vi "Open Camera.vi"(8 "error in (no error)":errorcluster) -> (0 "error out":errorcluster, 3 "Camera":refnum<data-value>)   [LabVIEW 2020, in "Test.Camera.lvclass"]
uses:
  Test.Camera.lvclass
  g_industrial_cam/Camera/Camera.lvclass
  Test.Camera.lvclass/Test.Camera.ctl
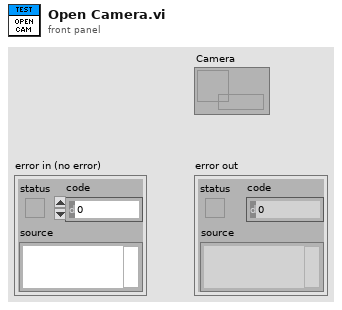
[diagram p1: front panel]
types:
  T1 = typedef "Device Enumeration.ctl" = cluster{"ID":string, "Protocol":string, "Vendor":string, "Model":string, "Serial":string, "Address":string}
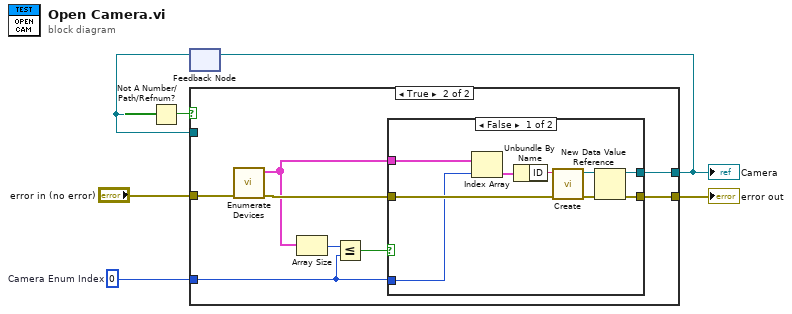
[diagram p0: block diagram]
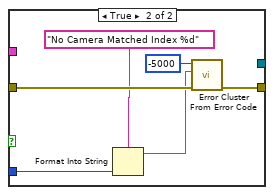
[diagram p3: hidden frame]
diagram:
  w1 = 0  # Camera Enum Index
  n1 = feedback #1() -> (w2:refnum<data-value>)  [unwired: 1 in]
  n2 = Not A Number/Path/Refnum?(number/path/refnum=w2) -> (NaN/Path/Refnum?=w3:bool)
  n3 = case shown="True" w3 {
    tunnel: "error in (no error)" -> [w8 w16]
    tunnel: [w8 w14] -> w5
    tunnel: [w7 w13] -> w4
    tunnel: w2 -> [w7 _]
    tunnel: w1 -> [_ w10]
    frame False {
    }
    frame True {
      n4 = call "Enumerate Devices.vi"("error in (no error)"=w16) -> ("error out"=w15:errorcluster, "Devices"=w12:T1[])  [unwired: 9 in]
      n5 = Array Size(array=w12) -> (size(s)=w11:i32)
      n6 = Less Or Equal?(x=w11, y=w10) -> (x <= y?=w9:bool)
      n7 = case shown="False" w9 {
        tunnel: w15 -> [w24 w31]
        tunnel: w10 -> [w22 w28]
        tunnel: [w20 w30] -> w14
        tunnel: [w18 _] -> w13
        tunnel: w12 -> [w17 _]
        frame False {
          n8 = Index Array(array=w17, index=w22) -> (element=w21:T1)
          n9 = Unbundle By Name(w21) -> ("ID"=w25:string)
          n10 = call "Create.vi"("error in (no error)"=w24, "Identifier (ID, IP etc)"=w25) -> ("error out"=w23:errorcluster, "Camera"=w19:refnum<class "Camera.lvclass">)  [unwired: 8 in]
          n11 = New Data Value Reference(data value=w19, error in=w23) -> (data value reference=w18:refnum<data-value>, error out=w20:errorcluster)
        }
        frame True {
          n12 = Format Into String(format string="No Camera Matched Index %d" ("error message (\"\")"), w28) -> (resulting string=w26:string)  [unwired: 2 in, 1 out]
          n13 = call <vilib>:"Error Cluster From Error Code.vi"("error in (no error)"=w31, "error message (\"\")"=w26, "error code (0)"=-5000) -> ("error out"=w30:errorcluster)  [unwired: 6 in]
        }
      }
    }
  }
  "error out" <- w5
  "Camera" <- w4
  n14 = feedback-in #1(w4) -> ()
